vi "TimeStringtoNumber.vi"(5 "time string":string) -> (0 "Total Seconds":dbl format="%.2f", 1 "Seconds":dbl format="%.2f", 2 "Minutes":i32, 3 "Hours":i32, 4 "Total mS":dbl format="%.2f")   [LabVIEW 2017]
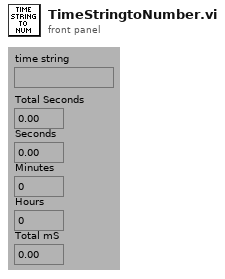
[diagram p1: front panel]
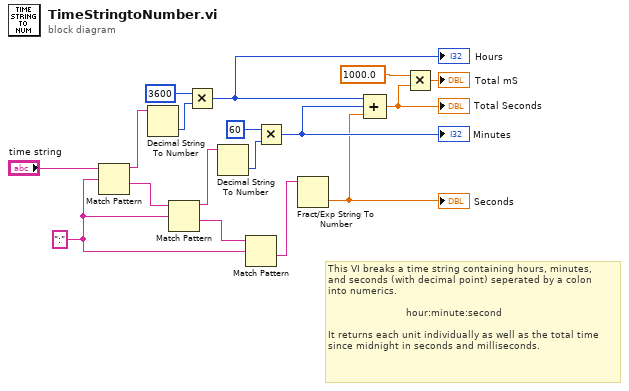
[diagram p0: block diagram]
diagram:
  w14 = ":" ("regular expression")
  # "This VI breaks a time string containing hours, minutes, \nand seconds (with decimal point) seperated by a colon \ninto numerics.\n  \n                          hour:minute:second\n\nIt returns each unit individually as well as the total time\nsince midnight in seconds and milliseconds."
  n1 = Match Pattern(string="time string", regular expression=w14) -> (before substring=w13:string, after substring=w16:string)  [unwired: 1 in, 2 out]
  n2 = Decimal String To Number(string=w13) -> (number=w11:i32)  [unwired: 2 in, 1 out]
  n3 = Match Pattern(string=w16, regular expression=w14) -> (before substring=w12:string, after substring=w15:string)  [unwired: 1 in, 2 out]
  n4 = Multiply(x=3600, y=w11) -> (x*y=w9:i32)
  "Hours" <- w9
  n5 = Decimal String To Number(string=w12) -> (number=w10:i32)  [unwired: 2 in, 1 out]
  n6 = Match Pattern(string=w15, regular expression=w14) -> (after substring=w1:string)  [unwired: 1 in, 3 out]
  n7 = Multiply(x=60, y=w10) -> (x*y=w8:i32)
  "Minutes" <- w8
  n8 = Fract/Exp String To Number(string=w1) -> (number=w7:dbl)  [unwired: 3 in, 1 out]
  "Seconds" <- w7
  n9 = Compound Arithmetic op=ADD(w9, w8, w7) -> (w2:dbl)
  "Total Seconds" <- w2
  n10 = Multiply(x=1000.0, y=w2) -> (x*y=→"Total mS":dbl)
